vi "eventos.vi"() -> ()   [LabVIEW 2011]
panel:
  in  "stop":bool
  out "Velocidad":i32(knob) scale=0.0..180.0
  in  "Reducir":bool
  in  "Aumentar":bool
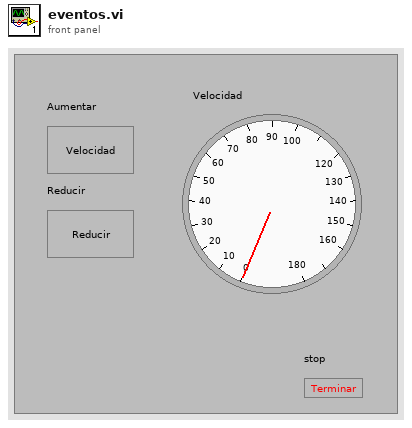
[diagram p1: front panel]
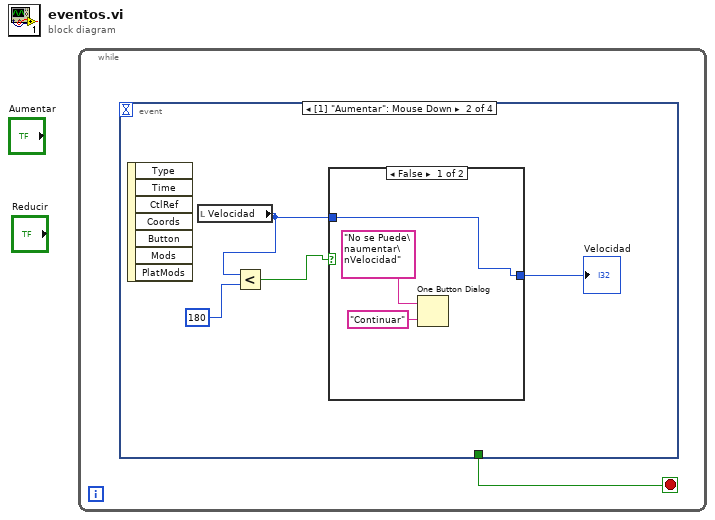
[diagram p0: block diagram]
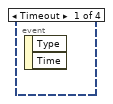
[diagram p2: hidden frame]
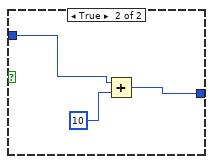
[diagram p3: hidden frame]
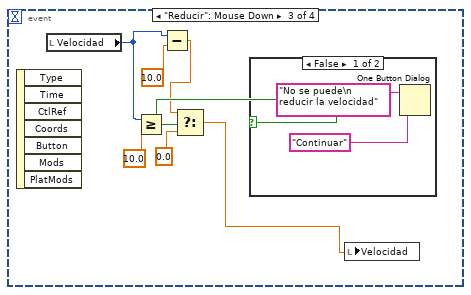
[diagram p4: hidden frame]
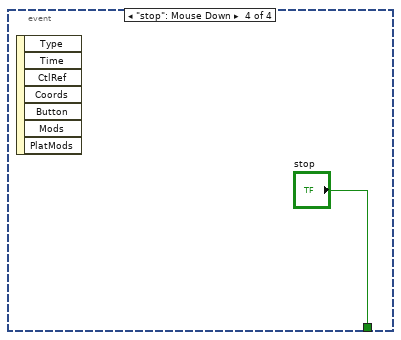
[diagram p6: hidden frame]
diagram:
  n1 = while {
    stop <- w1 stop-if-true
    n2 = event shown="[1] \"Aumentar\": Mouse Down" {
      selector: _ -> [_ _ _ _]
      dyn-events: _ -> [_ _ _ _]
      timeout: _ -> [_ _ _ _]
      tunnel: [_ _ _ "stop"] -> w1
      event Timeout {
        n3 = event-data() -> ()  [unwired: 1 in, 2 out]
      }
      event "Aumentar": Mouse Down {
        n4 = event-data() -> ()  [unwired: 1 in, 7 out]
        n5 = local read "Velocidad"() -> (w3:i32)
        n6 = Less?(x=w3, y=180) -> (x < y?=w4:bool)
        n7 = case shown="False" w4 {
          tunnel: w3 -> [w8 w11]
          tunnel: [w8 w9] -> w2
          frame False {
            n8 = One Button Dialog(message="No se Puede\naumentar\nVelocidad", button name ("OK")="Continuar") -> ()  [unwired: 1 out]
          }
          frame True {
            n9 = Add(x=w11, y=10) -> (x+y=w9:i32)
          }
        }
        "Velocidad" <- w2
      }
      event "Reducir": Mouse Down {
        n10 = event-data() -> ()  [unwired: 1 in, 7 out]
        n11 = local read "Velocidad"() -> (w13:i32)
        n12 = Greater Or Equal?(x=w13, y=10.0) -> (x >= y?=w16:bool)
        n13 = Subtract(x=w13, y=10.0) -> (x-y=w12:dbl)
        n14 = Select(t=w12, s=w16, f=0.0 ("y")) -> (s? t:f=w15:dbl)
        n15 = case shown="False" w16 {
          frame False {
            n16 = One Button Dialog(message="No se puede\n reducir la velocidad", button name ("OK")="Continuar") -> ()  [unwired: 1 out]
          }
          frame True {
          }
        }
        n17 = local write "Velocidad"(w15) -> ()
      }
      event "stop": Mouse Down {
        n18 = event-data() -> ()  [unwired: 1 in, 7 out]
      }
    }
  }
